vi "PXI-Enumerate DIO Lines.vi"() -> (8 "Lines":string[][](array[string]))   [LabVIEW 2020]
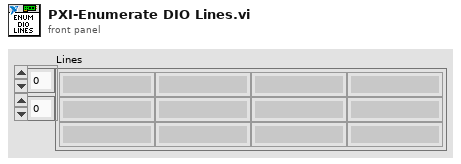
[diagram p1: front panel]
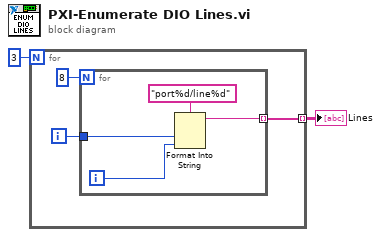
[diagram p0: block diagram]
diagram:
  n1 = for {
    N: 3 -> [_]
    tunnel: [w3] -> w1 mode=indexing
    i -> [w4]
    n2 = for {
      N: 8 -> [_]
      tunnel: w4 -> [w7]
      tunnel: [w6] -> w3 mode=indexing
      i -> [w8]
      n3 = Format Into String(format string="port%d/line%d", w7, w8) -> (resulting string=w6:string)  [unwired: 2 in, 1 out]
    }
  }
  "Lines" <- w1
